vi "Parse DB - 1553.vi"(0 "Path in":path=path "C:/work/SE/Opportunities/2012/Pilatus/201210/TestXMLs/Receiver.xml", 11 "error in (no error)":errorcluster) -> (4 "Bus":T1, 15 "error out":errorcluster)   [LabVIEW 2014, in "AIT 1553 Custom Device.lvlib"]
uses:
  AIT 1553 Custom Device.lvlib
  Controls/1553_Bus.ctl
  Controls/1553_Bus_Controller.ctl
  Controls/1553_BC_Message.ctl
  Controls/1553 Param.ctl
  Controls/1553_Acyclic_Frame.ctl
  Controls/1553_Bus_Monitor.ctl
  Controls/1553_BM_Message.ctl
  Controls/1553_RT_Message.ctl
  <userlib>/MIL-STD-1553/Owl1553.lvlib
  <vilib>/Utility/sysdir.llb/System Directory Type.ctl
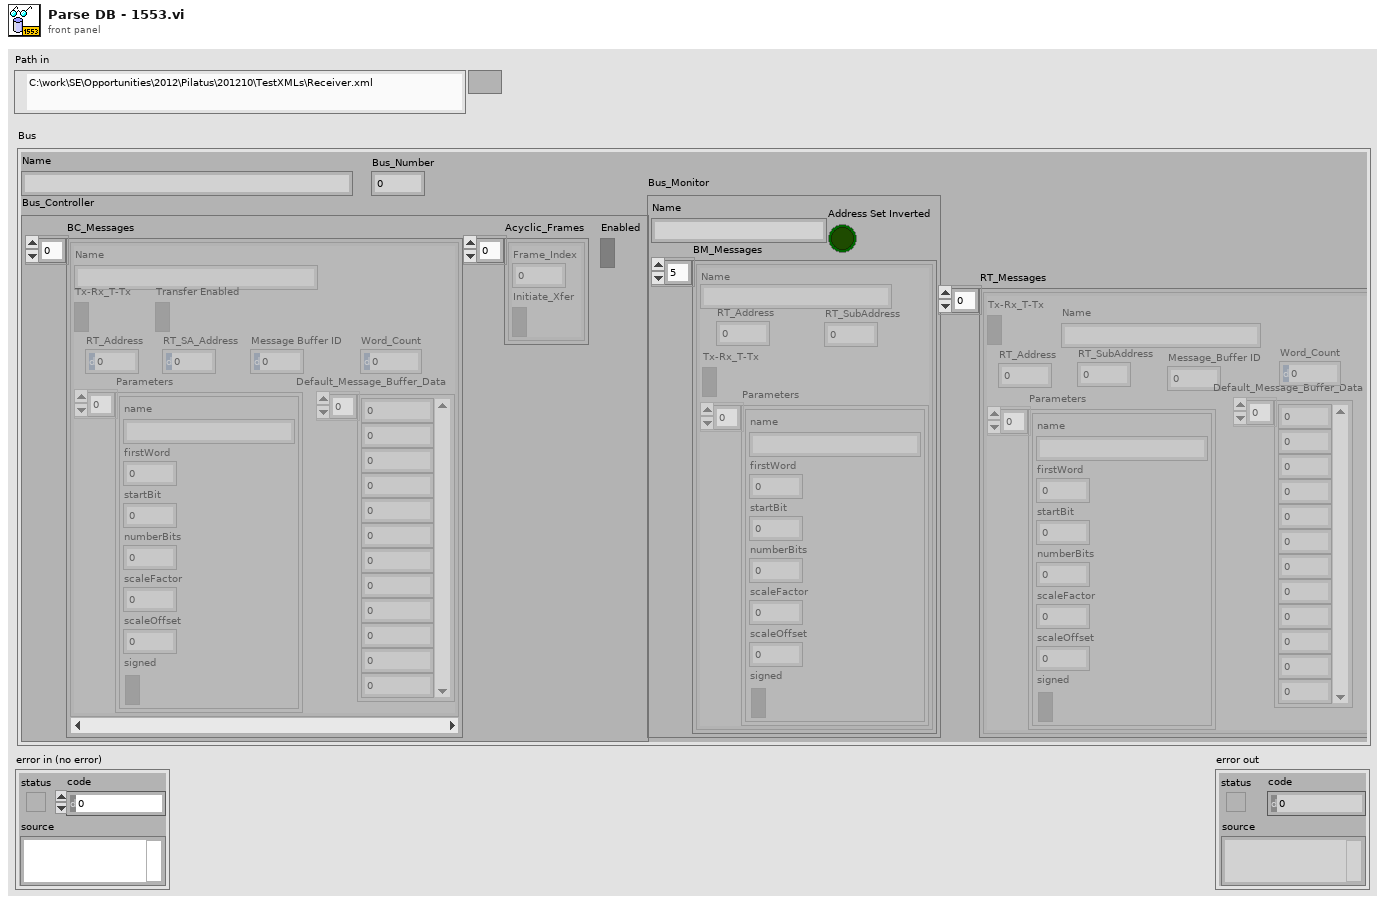
[diagram p1: front panel]
types:
  T1 = typedef "AIT 1553 Custom Device.lvlib/1553_Bus.ctl" = cluster{"Name":string, "Bus_Number":u8, "Bus_Controller":T2, "Bus_Monitor":T6, "RT_Messages":T8[]}
  T2 = typedef "AIT 1553 Custom Device.lvlib/1553_Bus_Controller.ctl" = cluster{"BC_Messages":T3[], "Acyclic_Frames":T5[], "Enabled":bool}
  T3 = typedef "AIT 1553 Custom Device.lvlib/1553_BC_Message.ctl" = cluster{"Name":string, "Tx-Rx_T-Tx":bool, "RT_Address":u8, "RT_SA_Address":u8, "Parameters":T4[], "Transfer Enabled":bool, "Message Buffer ID":u16, "Default_Message_Buffer_Data":u16[], "Word_Count":u8}
  T4 = typedef "AIT 1553 Custom Device.lvlib/1553 Param.ctl" = cluster{"name":string, "firstWord":i32, "startBit":i32, "numberBits":i32, "scaleFactor":dbl, "scaleOffset":dbl, "signed":bool}
  T5 = typedef "AIT 1553 Custom Device.lvlib/1553_Acyclic_Frame.ctl" = cluster{"Frame_Index":u8, "Initiate_Xfer":bool}
  T6 = typedef "AIT 1553 Custom Device.lvlib/1553_Bus_Monitor.ctl" = cluster{"Name":string, "BM_Messages":T7[], "Address Set Inverted":bool}
  T7 = typedef "AIT 1553 Custom Device.lvlib/1553_BM_Message.ctl" = cluster{"RT_Address":u8, "RT_SubAddress":u8, "Tx-Rx_T-Tx":bool, "Parameters":T4[], "Name":string}
  T8 = typedef "AIT 1553 Custom Device.lvlib/1553_RT_Message.ctl" = cluster{"RT_Address":u8, "RT_SubAddress":u8, "Tx-Rx_T-Tx":bool, "Parameters":T4[], "Message_Buffer ID":u16, "Default_Message_Buffer_Data":u16[], "Word_Count":u8, "Name":string}
  T9 = typedef "System Directory Type.ctl" = i32
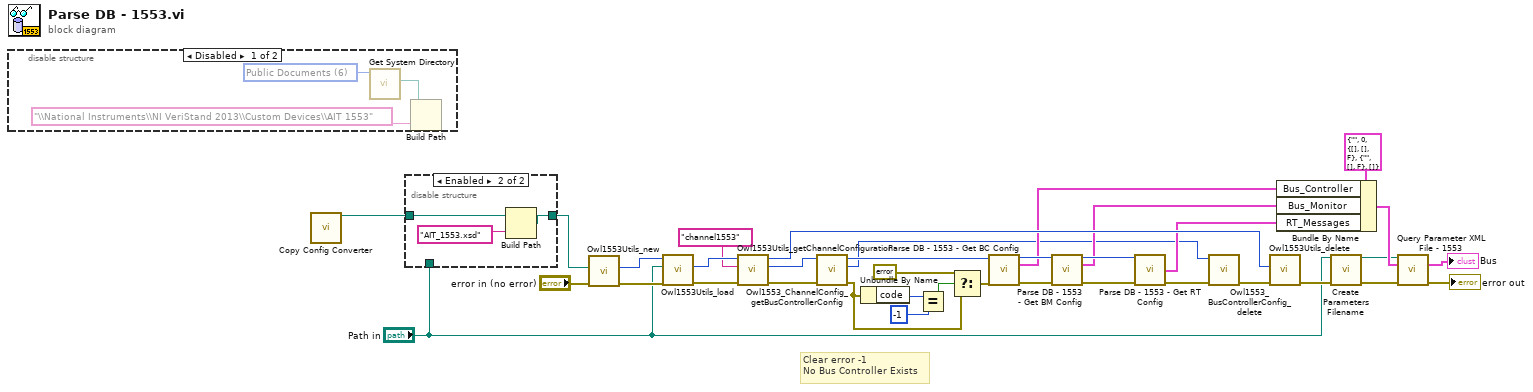
[diagram p0: block diagram]
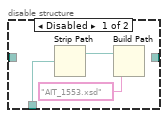
[diagram p3: hidden frame]
diagram:
  # "Clear error -1\nNo Bus Controller Exists"
  n1 = disable-structure shown="Disabled" {
    frame Disabled {
      w37 = T9 6 items=["User Home"=0, "User Desktop"=1, "User Documents"=2, "User Application Data"=3, "User Preferences"=4, "User Temporary"=5, "Public Documents"=6, "Public Application Data"=7, "Public Preferences"=8, "Public Cache"=13, "System Core Libraries"=9, "System Installed Libraries"=10, "Application Files"=11, "Boot Volume Root"=12] ("system directory type")
      n2 = call <vilib>:"Get System Directory.vi"("system directory type"=w37) -> ("system directory"=w38:path)  [unwired: 10 in]
      n3 = Build Path(base path=w38, name or relative path="\\National Instruments\\NI VeriStand 2013\\Custom Devices\\AIT 1553") -> ()  [unwired: 1 out]
    }
    frame Enabled {
    }
  }
  n4 = call "Copy Config Converter.vi"() -> ("original path to converter"=w1:path)  [unwired: 14 in, 1 out]
  n5 = disable-structure shown="Enabled" {
    disable-tunnel: "Path in" -> [w40 _]
    disable-tunnel: w1 -> [_ w45]
    disable-tunnel: [_ w43] -> w4
    frame Disabled {
      n6 = Strip Path(path=w40) -> (stripped path=w42:path)  [unwired: 1 out]
      n7 = Build Path(base path=w42, name or relative path="AIT_1553.xsd") -> ()  [unwired: 1 out]
    }
    frame Enabled {
      n8 = Build Path(base path=w45, name or relative path="AIT_1553.xsd") -> (appended path=w43:path)
    }
  }
  n9 = call <userlib>:"Owl1553Utils_new.vi"("error in (no error)"="error in (no error)", "Xml Schema Path in"=w4) -> ("error out"=w36:errorcluster, "xml config handle"=w33:u64)  [unwired: 8 in]
  n10 = call <userlib>:"Owl1553Utils_load.vi"("error in (no error)"=w36, "Path in"="Path in", "xml config handle"=w33) -> ("error out"=w35:errorcluster, "xml config handle"=w34:u64)  [unwired: 7 in]
  n11 = call <userlib>:"Owl1553Utils_getChannelConfiguration.vi"("error in (no error)"=w35, "X Path"="channel1553", "xml config handle"=w34) -> ("error out"=w13:errorcluster, "channel config handle"=w27:u64, "xml config handle"=w26:u64)  [unwired: 6 in]
  n12 = call <userlib>:"Owl1553_ChannelConfig_getBusControllerConfig.vi"("error in (no error)"=w13, "channel config handle"=w27) -> ("error out"=w9:errorcluster, "bus controller config handle"=w20:u64, "channel config handle"=w28:u64)  [unwired: 7 in]
  n13 = Unbundle By Name(w9) -> ("code"=w12:i32)
  n14 = Equal?(x=w12, y=-1) -> (x = y?=w5:bool)
  n15 = Select(t=errorcluster {"status"=FALSE, "code"=0, "source"=""} ("error in (no error)"), s=w5, f=w9) -> (s? t:f=w8:errorcluster)
  n16 = call "Parse DB - 1553 - Get BC Config.vi"("channel config handle"=w28, "error in (no error)"=w8) -> ("channel config handle out"=w30:u32, "Bus_Controller"=w23:T2, "error out"=w7:errorcluster)  [unwired: 10 in, 1 out]
  n17 = call "Parse DB - 1553 - Get BM Config.vi"("channel config handle"=w30, "error in (no error)"=w7) -> ("channel config handle out"=w29:u32, "Bus_Monitor"=w22:T6, "error out"=w6:errorcluster)  [unwired: 10 in, 1 out]
  n18 = call "Parse DB - 1553 - Get RT Config.vi"("channel config handle"=w29, "error in (no error)"=w6) -> ("RT_Messages"=w21:T8[], "error out"=w25:errorcluster)  [unwired: 11 in, 1 out]
  n19 = call <userlib>:"Owl1553_BusControllerConfig_delete.vi"("error in (no error)"=w25, "bus controller config handle"=w20) -> ("error out"=w32:errorcluster)  [unwired: 9 in]
  n20 = call <userlib>:"Owl1553Utils_delete.vi"("error in (no error)"=w32, "xml config handle"=w26) -> ("error out"=w17:errorcluster)  [unwired: 9 in]
  n21 = Bundle By Name(cluster=T1 {"Name"="", "Bus_Number"=0, "Bus_Controller"={"BC_Messages"=[], "Acyclic_Frames"=[], "Enabled"=FALSE}, "Bus_Monitor"={"Name"="", "BM_Messages"=[], "Address Set Inverted"=FALSE}, "RT_Messages"=[]} ("Bus"), "Bus_Controller"=w23, "Bus_Monitor"=w22, "RT_Messages"=w21) -> (w18:T1)
  n22 = call "Create Parameters Filename.vi"("Simulyzer File Path"="Path in", "error in (no error)"=w17) -> ("Parm File Path"=w14:path, "error out"=w15:errorcluster)  [unwired: 12 in]
  n23 = call "Query Parameter XML File - 1553.vi"("Path in"=w14, "Bus Without Parms"=w18, "error in (no error)"=w15) -> ("Bus With Parms"=→"Bus":T1, "error out"=→"error out":errorcluster)  [unwired: 11 in]
